vi "Image Server Loop.vi"(8 "error in (no error)":errorcluster, 11 "Image Notifier":refnum<notifier>) -> ()   [LabVIEW 2015]
doc: "This VI is used to send images to the dashboard using the second enet port on the 8 slot controller. This is provided for compatibility, but is higher overhead than using the Camera MJPG approach.\n\nThis software is licensed. Open the labview\\readme\\WPI Robotics Library Open Source License.txt file for more information."
uses:
  <vilib>/Rock Robotics/SystemInterfaces/NetworkCommunication/NetComm_UsageReport_ResourceType.ctl
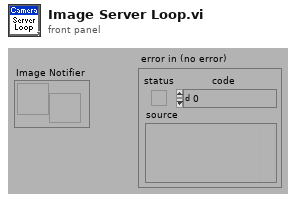
[diagram p1: front panel]
types:
  T1 = cluster{"fps":i32, "compression":i32, "compression 2":i32}
  T2 = typedef "NetComm_UsageReport_ResourceType.ctl" = enum8{"Controller", "Module", "Language", "CANPlugin", "Accelerometer", "ADXL345", "AnalogChannel", "AnalogTrigger", "AnalogTriggerOutput", "CANJaguar", "Compressor", "Counter", "Dashboard", "DigitalInput", "DigitalOutput", "DriverStationCIO", "DriverStationEIO", "DriverStationLCD", "Encoder", "GearTooth", "Gyro", "I2C", "Framework", "Jaguar", "Joystick", "Kinect", "KinectStick", "PIDController", "Preferences", "PWM", "Relay", "RobotDrive", "SerialPort", "Servo", "Solenoid", "SPI", "Task", "Ultrasonic", "Victor", "Button", "Command", "AxisCamera", "PCVideoServer", "SmartDashboard", "Talon", "HiTechnicColorSensor", "HiTechnicAccel", "HiTechnicCompass", "SRF08", "AnalogOutput", "Victor SP", "Talon SRX", "CAN Talon SRX", "ADXL362 Accel", "ADXRS450 Gyro", "Rev SPARK", "Mindsensors SD540", "Digital Filter"}
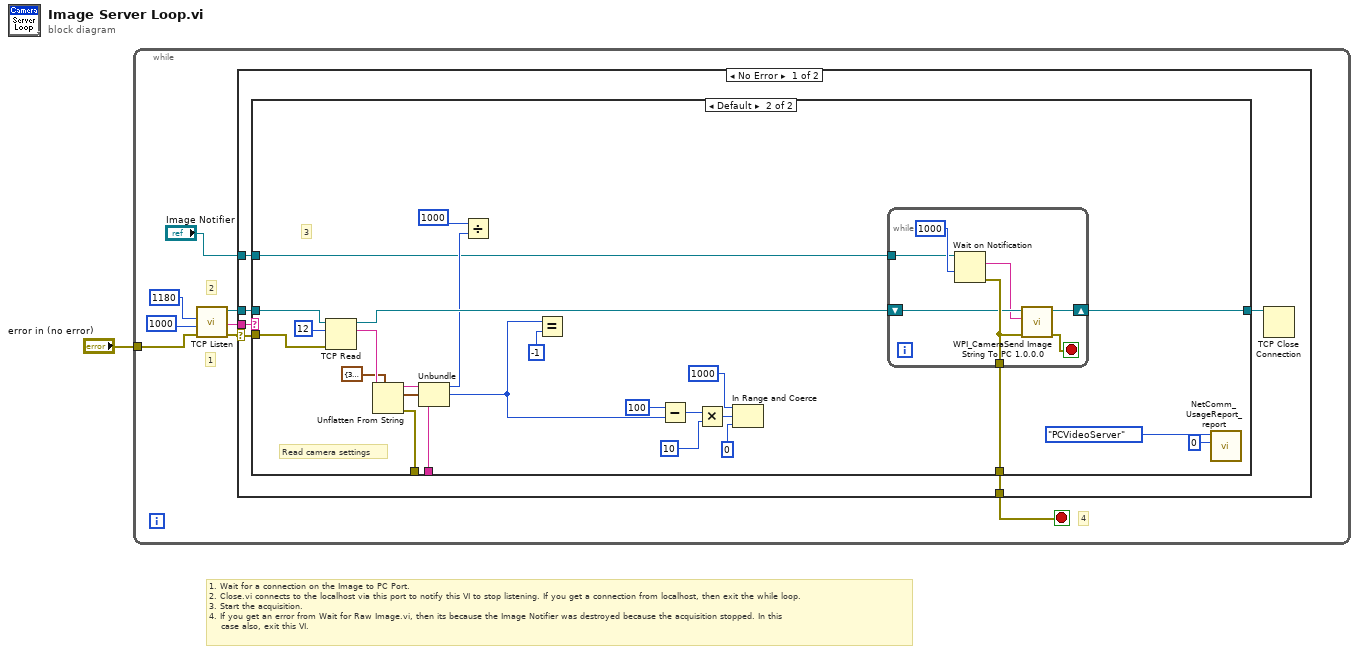
[diagram p0: block diagram]
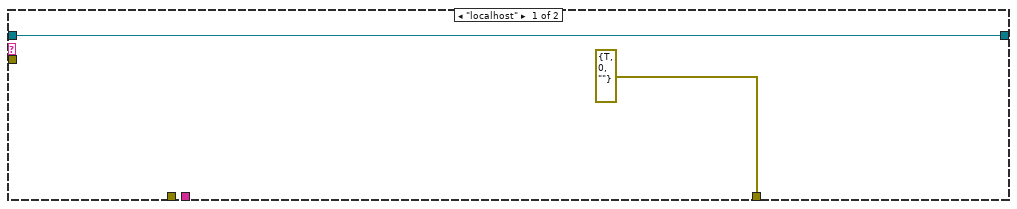
[diagram p2: hidden frame]
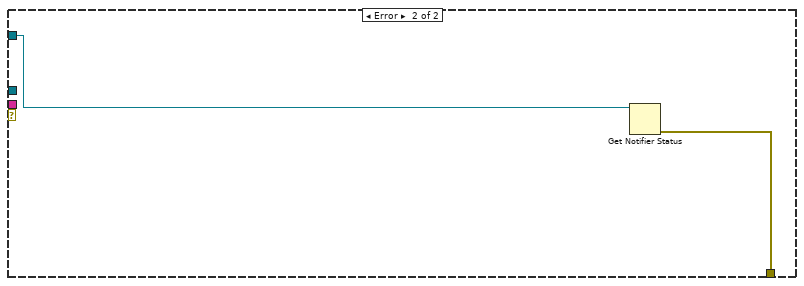
[diagram p3: hidden frame]
diagram:
  # "1. Wait for a connection on the Image to PC Port.\n2. Close.vi connects to the localhost via this port to notify this VI to stop listening. If you get a connection from localhost, then exit the while loop.\n3. Start the acquisition.\n4. If you get an error from Wait for Raw Image.vi, then its because the Image Notifier was destroyed because the acquisition stopped. In this\n    case also, exit this VI."
  n1 = while {
    tunnel: "error in (no error)" -> [w8]
    stop <- w6 stop-if-true
    # "4"
    # "1"
    # "2"
    n2 = call <vilib>:"TCP Listen.vi"("error in (no error)"=w8, "timeout ms (wait forever: -1)"=u16 1000 ("port"), "port"=u16 1180) -> ("error out"=w4:errorcluster, "remote address"=w9:string, "connection ID"=w7:refnum<k5>)  [unwired: 1 in, 5 out]
    n3 = case shown="No Error" w4 {
      selector: w4 -> [w11 _]
      tunnel: w9 -> [w15 _]
      tunnel: w7 -> [w14 _]
      tunnel: [w13 w50] -> w6
      tunnel: "Image Notifier" -> [w10 w49]
      frame No Error {
        n4 = case shown="Default" w15 {
          tunnel: w11 -> [_ w33]
          tunnel: w14 -> [w16 w37]
          tunnel: [errorcluster {"status"=TRUE, "code"=0, "source"=""} ("error out 2") w41] -> w13
          tunnel: [w16 w40] -> w12
          tunnel: [_ w20] -> _
          tunnel: [_ w19] -> _
          tunnel: w10 -> [_ w18]
          frame "localhost" {
          }
          frame Default {
            # "Read camera settings"
            # "3"
            n5 = TCP Read(connection ID=w37, bytes to read=12, error in (no error)=w33) -> (connection ID out=w36:refnum<k5>, data out=w34:string)  [unwired: 2 in, 1 out]
            n6 = Unflatten From String(type=T1 {"fps"=30, "compression"=32, "compression 2"=32} ("Camera Settings"), binary string=w34) -> (rest of the binary string=w19:string, value=w32:T1, error out=w20:errorcluster)  [unwired: 3 in]
            n7 = Unbundle(w32) -> ("fps"=w30:i32, "compression"=w21:i32)  [unwired: 1 out]
            n8 = Divide(x=u16 1000 ("port"), y=w30) -> ()  [unwired: 1 out]
            n9 = Equal?(x=w21, y=-1) -> ()  [unwired: 1 out]
            n10 = Subtract(x=100, y=w21) -> (x-y=w25:i32)
            n11 = Multiply(x=w25, y=10) -> (x*y=w27:i32)
            n12 = In Range and Coerce(upper limit=1000, x=w27, lower limit=0) -> ()  [unwired: 2 out]
            n13 = while {
              tunnel: [w48] -> w41
              shift-right: [w47] -> w40
              shift-left: w36 -> [w46]
              tunnel: w18 -> [w43]
              stop <- w42 stop-if-true
              n14 = Wait on Notification(notifier=w43, timeout in ms (-1)=1000 ("Timeout in ms (-1)")) -> (notification=w45:string, error out=w48:errorcluster)  [unwired: 1 in, 3 out]
              n15 = call <vilib>:"WPI_CameraSend Image String To PC 1.0.0.0.vi"("error in (no error)"=w48, "String"=w45, "TCP Connection ID"=w46) -> ("error out"=w42:errorcluster, "TCP Connection ID out"=w47:refnum<k5>)  [unwired: 7 out]
            }
            n16 = call <vilib>:"NetComm_UsageReport_report.vi"("Instance Number"=u8 0, "Resource Type"=NetComm_UsageReport_ResourceType."PCVideoServer") -> ()  [unwired: 10 in]
          }
        }
        n17 = TCP Close Connection(connection ID=w12) -> ()  [unwired: 1 in, 3 out]
      }
      frame Error {
        n18 = Get Notifier Status(notifier=w49) -> (error out=w50:errorcluster)  [unwired: 1 in, 4 out]
      }
    }
  }
